vi "LQG_Target.vi"   [LabVIEW 2022 SP3]
uses:
  <vilib>/rvi/interface/RandomDataEmulation/niFpgaRandomDataHandleErrors.vi
  <vilib>/rvi/DataTransferAndStorage/Container/XNode/niFpgaContainer.xnode
  <vilib>/rvi/interface/RandomDataEmulation/nirviRandomDataFpgaReadWriteTemplate.vi
  <vilib>/rvi/linearAlgebra/MatrixMultiply/XNode/nifxpla_MatrixMultiply.xnode
  <vilib>/rvi/linearAlgebra/MatrixMultiply/simVIs/nifxpla_MatrixMultiply_SimTemplateEinEout.vi
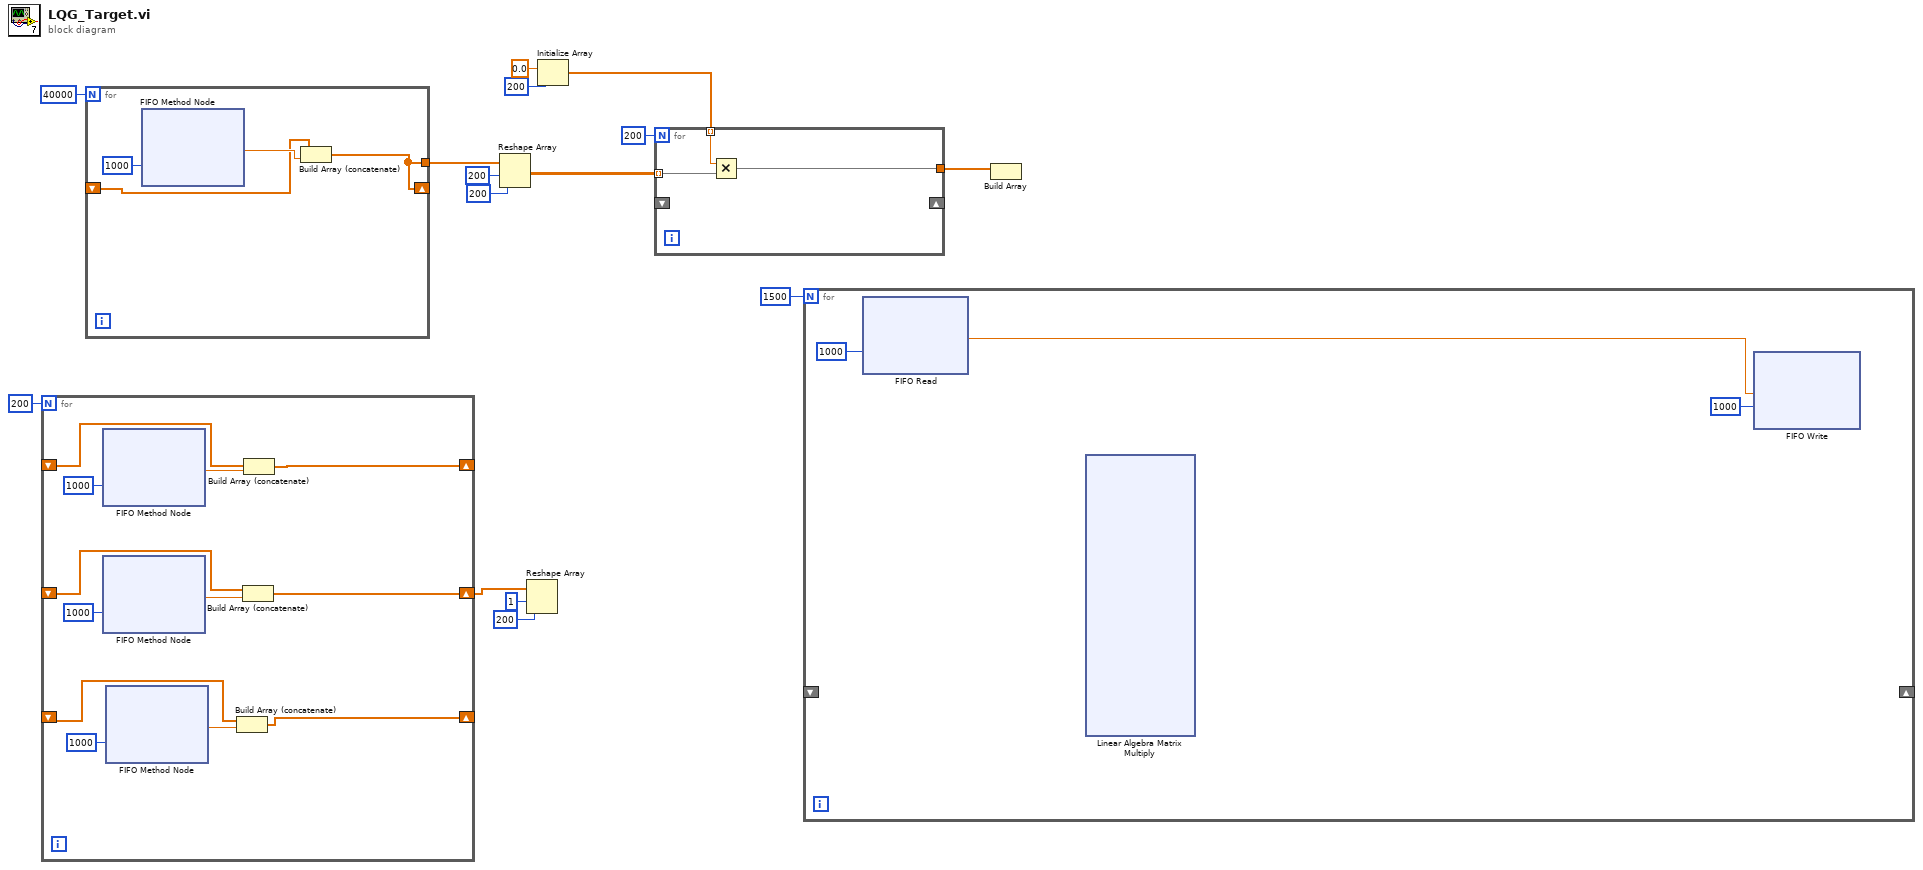
[diagram p0: block diagram]
diagram:
  n1 = for {
    N: 200 -> [_]
    shift-right: [w20] -> _
    shift-left: _ -> [w19]
    shift-right: [w17] -> w9
    shift-left: _ -> [w18]
    shift-right: [w21] -> _
    shift-left: _ -> [w16]
    n2 = xnode ("FIFO Method Node")("Timeout"=1000) -> ("Element"=w24:sgl)  [unwired: 1 in, 2 out]
    n3 = xnode ("FIFO Method Node")("Timeout"=1000) -> ("Element"=w23:sgl)  [unwired: 1 in, 2 out]
    n4 = xnode ("FIFO Method Node")("Timeout"=1000) -> ("Element"=w22:sgl)  [unwired: 1 in, 2 out]
    n5 = Build Array (concatenate)(w19, w22) -> (w20:sgl[])
    n6 = Build Array (concatenate)(w18, w23) -> (w17:sgl[])
    n7 = Build Array (concatenate)(w16, w24) -> (w21:sgl[])
  }
  n8 = for {
    N: 40000 -> [_]
    shift-right: [w29] -> _
    shift-left: _ -> [w28]
    tunnel: [w29] -> w13
    n9 = xnode ("FIFO Method Node")("Timeout"=1000) -> ("Element"=w30:sgl)  [unwired: 1 in, 2 out]
    n10 = Build Array (concatenate)(w28, w30) -> (w29:sgl[])
  }
  n11 = Reshape Array(w13, 200 ("dimension size"), 200 ("dimension size")) -> (w2:sgl[][])
  n12 = Reshape Array(w9, 1 ("dimension size"), 200 ("dimension size")) -> ()  [unwired: 1 out]
  n13 = Initialize Array(sgl 0.0 ("element"), 200 ("dimension size")) -> (w3:sgl[])
  n14 = for {
    N: 200 -> [_]
    tunnel: w3 -> [w34] mode=indexing
    tunnel: w2 -> [w33] mode=indexing
    shift-right: _ -> [_]
    shift-left: _ -> [_]
    tunnel: [w32] -> w1
    n15 = Multiply(x=w34, y=w33) -> (x*y=w32:sgl[])
  }
  n16 = for {
    N: 1500 -> [_]
    shift-right: _ -> [_]
    shift-left: _ -> [_]
    n17 = xnode ("FIFO Read")("Timeout"=1000) -> ("Element"=w35:sgl)  [unwired: 1 in, 2 out]
    n18 = xnode "Linear Algebra Matrix Multiply"() -> ()  [unwired: 7 in, 6 out]
    n19 = xnode ("FIFO Write")("Element"=w35, "Timeout"=1000) -> ()  [unwired: 1 in, 2 out]
  }
  n20 = Build Array(w1) -> ()  [unwired: 1 in, 1 out]
